vi "Autonomous Independent.vi"() -> ()   [LabVIEW 2012]
doc: "This VI is called when autonomous begins, and will automatically be terminated when autonomous ends. You can carry out timed or sensor driven robot movement independently without needing to return to the caller."
uses:
  Robot Global Data.vi
panel:
  out "x <= y?":bool
  out "x .or. y?":bool
  # "Be sure to right-click and choose Data Operations>>Make Current Value default if you want to save the array values with the VI"
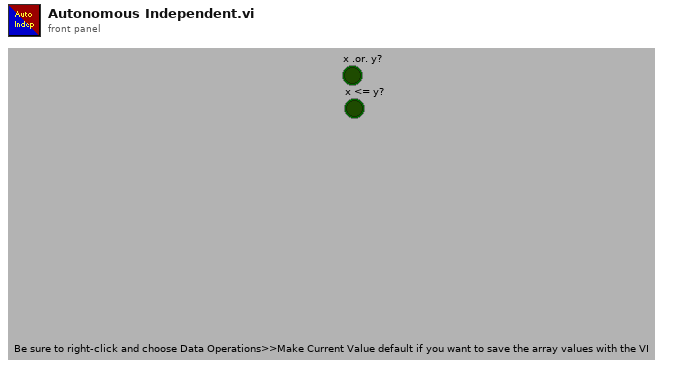
[diagram p1: front panel]
types:
  T1 = typedef "WPI_DigitalInputDevRef.ctl" = cluster{"DevStatus":errorcluster, "DIO Channel":T2, "Digital Module":T3}
  T2 = typedef "FPGA_DIOChannel.ctl" = enum8{"DIO 1", "DIO 2", "DIO 3", "DIO 4", "DIO 5", "DIO 6", "DIO 7", "DIO 8", "DIO 9", "DIO 10", "DIO 11", "DIO 12", "DIO 13", "DIO 14", "Invalid"}
  T3 = typedef "FPGA_TypedefDigitalModule.ctl" = enum16{"Digital Module 1", "Digital Module 2"}
  T4 = cluster{"Frisbee_Catch":bool, "Shooter_Ready":bool, "LeadScrewEnd":bool}
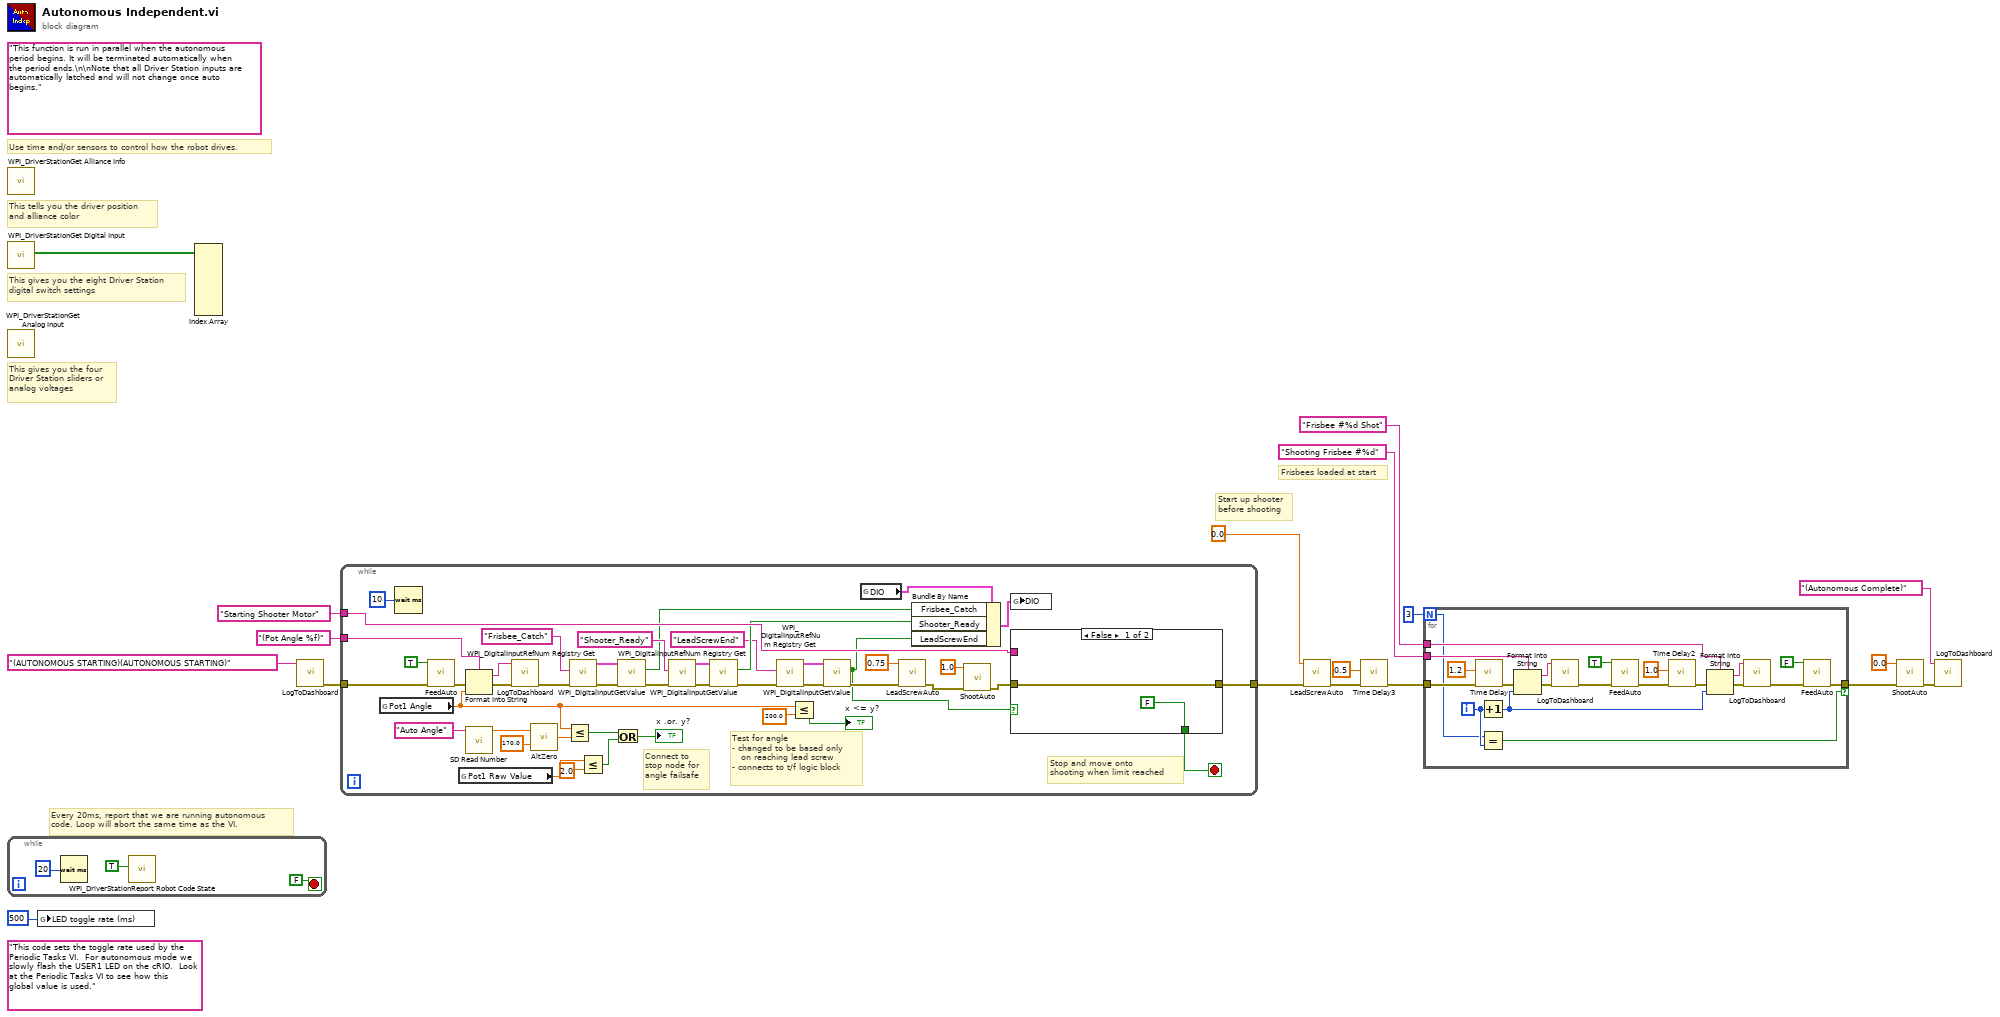
[diagram p0: block diagram]
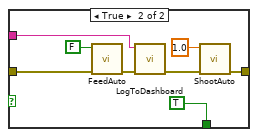
[diagram p2: hidden frame]
diagram:
  (unwired) "This code sets the toggle rate used by the Periodic Tasks VI.  For autonomous mode we slowly flash the USER1 LED on the cRIO.  Look at the Periodic Tasks VI to see how this global value is used."
  (unwired) "This function is run in parallel when the autonomous period begins. It will be terminated automatically when the period ends.\n\nNote that all Driver Station inputs are automatically latched and will not change once auto begins."
  # "Start up shooter\nbefore shooting"
  # "Frisbees loaded at start"
  # "Every 20ms, report that we are running autonomous\ncode. Loop will abort the same time as the VI."
  # "Use time and/or sensors to control how the robot drives."
  # "This tells you the driver position\nand alliance color"
  # "This gives you the eight Driver Station\ndigital switch settings"
  # "This gives you the four\nDriver Station sliders or\nanalog voltages"
  n1 = call <vilib>:"WPI_DriverStationGet Alliance Info.vi"() -> ()  [unwired: 12 out]
  n2 = call <vilib>:"WPI_DriverStationGet Digital Input.vi"() -> ("Driver Station Digital Input (1-8)"=w18:bool[])  [unwired: 11 out]
  n3 = call <vilib>:"WPI_DriverStationGet Analog Input.vi"() -> ()  [unwired: 12 out]
  n4 = while {
    stop <- FALSE stop-if-true
    n5 = Wait (ms)(milliseconds to wait=u32 20) -> ()  [unwired: 1 out]
    n6 = call <vilib>:"WPI_DriverStationReport Robot Code State.vi"("Autonomous"=TRUE) -> ()  [unwired: 10 in, 1 out]
  }
  n7 = global write "Robot Global Data.vi" "LED toggle rate (ms)"(u32 500 ("LED ms toggle rate")) -> ()
  n8 = Index Array(array=w18) -> ()  [unwired: 8 in, 8 out]
  n9 = call "LogToDashboard.vi"("Info"="(AUTONOMOUS STARTING)(AUTONOMOUS STARTING)" ("line text")) -> ("error out"=w7:errorcluster)  [unwired: 10 in]
  n10 = while {
    tunnel: "(Pot Angle %f)" -> [w63]
    tunnel: w7 -> [w35]
    tunnel: "Starting Shooter Motor" ("line text") -> [w59]
    tunnel: [w57] -> w5
    stop <- w25 stop-if-true
    # "Stop and move onto\nshooting when limit reached"
    # "Connect to\nstop node for\nangle failsafe"
    # "Test for angle\n- changed to be based only\n   on reaching lead screw\n- connects to t/f logic block"
    n11 = global read "Robot Global Data.vi" "Pot1 Angle"() -> (w61:dbl)
    n12 = Wait (ms)(milliseconds to wait=u32 10) -> ()  [unwired: 1 out]
    n13 = call "FeedAuto.vi"("error in (no error)"=w35, "Feed"=TRUE) -> ("error out"=w34:errorcluster)  [unwired: 9 in]
    n14 = global read "Robot Global Data.vi" "Pot1 Raw Value"() -> (w39:dbl)
    n15 = Format Into String(format string=w63, error in=w34, w61) -> (resulting string=w64:string, error out=w62:errorcluster)  [unwired: 1 in]
    n16 = call <vilib>:"SD Read Number.vi"("Name"="Auto Angle") -> ("Numeric"=w30:dbl)  [unwired: 8 in, 2 out]
    n17 = call "LogToDashboard.vi"("error in (no error)"=w62, "Info"=w64) -> ("error out"=w40:errorcluster)  [unwired: 9 in]
    n18 = call "AltZero.vi"("z"=170.0, "x"=w30) -> ("y"=w31:dbl)
    n19 = Less Or Equal?(x=w61, y=w31) -> (x <= y?=w36:bool)
    n20 = call <vilib>:"WPI_DigitalInputRefNum Registry Get.vi"("error in (no error)"=w40, "refnum name"="Frisbee_Catch") -> ("error out"=w49:errorcluster, "DigitalInputDevRef"=w50:T1)  [unwired: 8 in]
    n21 = Less Or Equal?(x=w39, y=2.0) -> (x <= y?=w37:bool)
    n22 = Or(x=w36, y=w37) -> (x .or. y?=→"x .or. y?":bool)
    n23 = call <vilib>:"WPI_DigitalInputGetValue.vi"("error in (no error)"=w49, "DigitalInputDevRef"=w50) -> ("error out"=w42:errorcluster, "Value"=w44:bool)  [unwired: 7 in, 1 out]
    n24 = call <vilib>:"WPI_DigitalInputRefNum Registry Get.vi"("error in (no error)"=w42, "refnum name"="Shooter_Ready") -> ("error out"=w52:errorcluster, "DigitalInputDevRef"=w51:T1)  [unwired: 8 in]
    n25 = call <vilib>:"WPI_DigitalInputGetValue.vi"("error in (no error)"=w52, "DigitalInputDevRef"=w51) -> ("error out"=w43:errorcluster, "Value"=w48:bool)  [unwired: 7 in, 1 out]
    n26 = call <vilib>:"WPI_DigitalInputRefNum Registry Get.vi"("error in (no error)"=w43, "refnum name"="LeadScrewEnd") -> ("error out"=w46:errorcluster, "DigitalInputDevRef"=w45:T1)  [unwired: 8 in]
    n27 = Less Or Equal?(x=w61, y=200.0) -> (x <= y?=→"x <= y?":bool)
    n28 = call <vilib>:"WPI_DigitalInputGetValue.vi"("error in (no error)"=w46, "DigitalInputDevRef"=w45) -> ("error out"=w41:errorcluster, "Value"=w26:bool)  [unwired: 7 in, 1 out]
    n29 = global read "Robot Global Data.vi" "DIO"() -> (w56:T4)
    n30 = call "LeadScrewAuto.vi"("error in (no error)"=w41, "LeadScrew"=0.75 ("Output")) -> ("error out"=w24:errorcluster)  [unwired: 9 in]
    n31 = Bundle By Name(cluster=w56, "Frisbee_Catch"=w44, "Shooter_Ready"=w48, "LeadScrewEnd"=w26) -> (w55:T4)
    n32 = call "ShootAuto.vi"("error in (no error)"=w24, "Shooter"=1.0) -> ("error out"=w23:errorcluster)  [unwired: 9 in]
    n33 = global write "Robot Global Data.vi" "DIO"(w55) -> ()
    n34 = case shown="False" w26 {
      tunnel: w59 -> [_ w75]
      tunnel: w23 -> [w67 w71]
      tunnel: [w67 w74] -> w57
      tunnel: [FALSE TRUE] -> w25
      frame False {
      }
      frame True {
        n35 = call "FeedAuto.vi"("error in (no error)"=w71, "Feed"=FALSE) -> ("error out"=w70:errorcluster)  [unwired: 9 in]
        n36 = call "LogToDashboard.vi"("error in (no error)"=w70, "Info"=w75) -> ("error out"=w72:errorcluster)  [unwired: 9 in]
        n37 = call "ShootAuto.vi"("error in (no error)"=w72, "Shooter"=1.0 ("Output")) -> ("error out"=w74:errorcluster)  [unwired: 9 in]
      }
    }
  }
  n38 = call "LeadScrewAuto.vi"("error in (no error)"=w5, "LeadScrew"=0.0) -> ("error out"=w6:errorcluster)  [unwired: 9 in]
  n39 = call "Time Delay3"("error in (no error)"=w6, "Delay Time (s)"=0.5) -> ("error out"=w12:errorcluster)  [unwired: 9 in]
  n40 = for {
    N: 3 -> [w87]
    tunnel: w12 -> [w96]
    tunnel: "Shooting Frisbee #%d" -> [w92]
    tunnel: "Frisbee #%d Shot" -> [w88]
    tunnel: [w84] -> w3 if=w82
    i -> [w91]
    n41 = call "Time Delay"("error in (no error)"=w96, "Delay Time (s)"=1.2) -> ("error out"=w77:errorcluster)  [unwired: 9 in]
    n42 = Increment(x=w91) -> (x+1=w90:i32)
    n43 = Equal?(x=w87, y=w91) -> (x = y?=w82:bool)
    n44 = Format Into String(format string=w92, error in=w77, w90) -> (resulting string=w93:string, error out=w78:errorcluster)  [unwired: 1 in]
    n45 = call "LogToDashboard.vi"("error in (no error)"=w78, "Info"=w93) -> ("error out"=w80:errorcluster)  [unwired: 9 in]
    n46 = call "FeedAuto.vi"("error in (no error)"=w80, "Feed"=TRUE) -> ("error out"=w79:errorcluster)  [unwired: 9 in]
    n47 = call "Time Delay2"("error in (no error)"=w79, "Delay Time (s)"=1.0) -> ("error out"=w83:errorcluster)  [unwired: 9 in]
    n48 = Format Into String(format string=w88, error in=w83, w90) -> (resulting string=w89:string, error out=w76:errorcluster)  [unwired: 1 in]
    n49 = call "LogToDashboard.vi"("error in (no error)"=w76, "Info"=w89) -> ("error out"=w85:errorcluster)  [unwired: 9 in]
    n50 = call "FeedAuto.vi"("error in (no error)"=w85, "Feed"=FALSE) -> ("error out"=w84:errorcluster)  [unwired: 9 in]
  }
  n51 = call "ShootAuto.vi"("error in (no error)"=w3, "Shooter"=0.0 ("LeadScrew")) -> ("error out"=w1:errorcluster)  [unwired: 9 in]
  n52 = call "LogToDashboard.vi"("error in (no error)"=w1, "Info"="(Autonomous Complete)" ("line text")) -> ()  [unwired: 9 in, 1 out]
